vi "Parametri ADC.vi"() -> ()   [LabVIEW 2021]
uses:
  <vilib>/measure/madcrms.llb/Basic Averaged DC-RMS for 1 Chan.vi
  <vilib>/express/express analysis/Spectral/Block/exnSpectralBlock spectral measurements RMS poly.vi
  <vilib>/express/express analysis/Spectral/Block/exnSpectralBlock spectral measurements RMS DDT.vi
  <vilib>/express/express analysis/Spectral/XNode/ExpressSpectralMeasurementsBlockNode.xnode
  <vilib>/measure/NI_MAPro.lvlib
panel:
  out "Frequenza fondamentale":dbl
  out "ENOB ideale":dbl
  out "df":dbl
  out "Ampiezza fondamentale":dbl
  out "THD (db)":dbl
  out "ENOB (corretto rispetto al full scale)":dbl
  out "SINAD(db)":dbl
  out "SNR(db)":dbl
  out "DFT (dB)":dynamicdata(graph)
  out "numero punti dft":i32
  out "Ampiezza":dbl
  out "Frequenza":dbl
  out "SFDR":dbl
  out "DFT (lineare)":dynamicdata(graph)
  out "Segnale acquisito":dynamicdata(graph)
  # "distanza tra un punto\n della dft e il successivo"
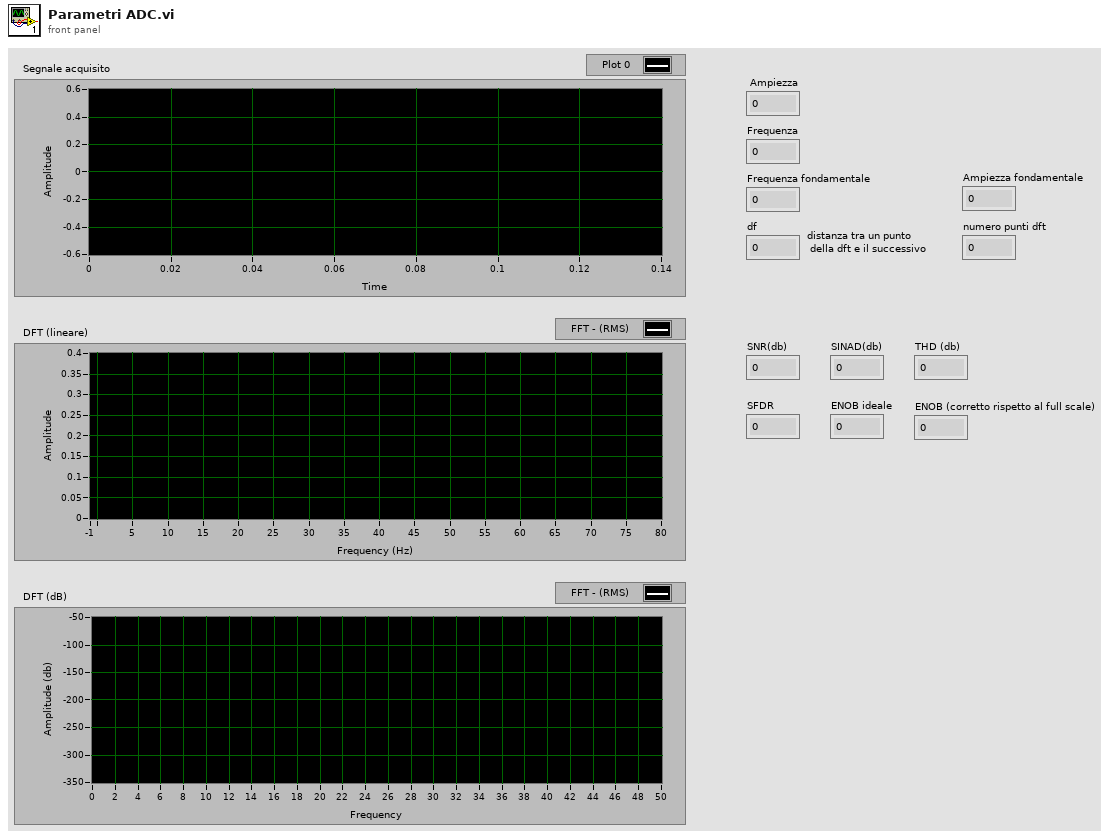
[diagram p1: front panel]
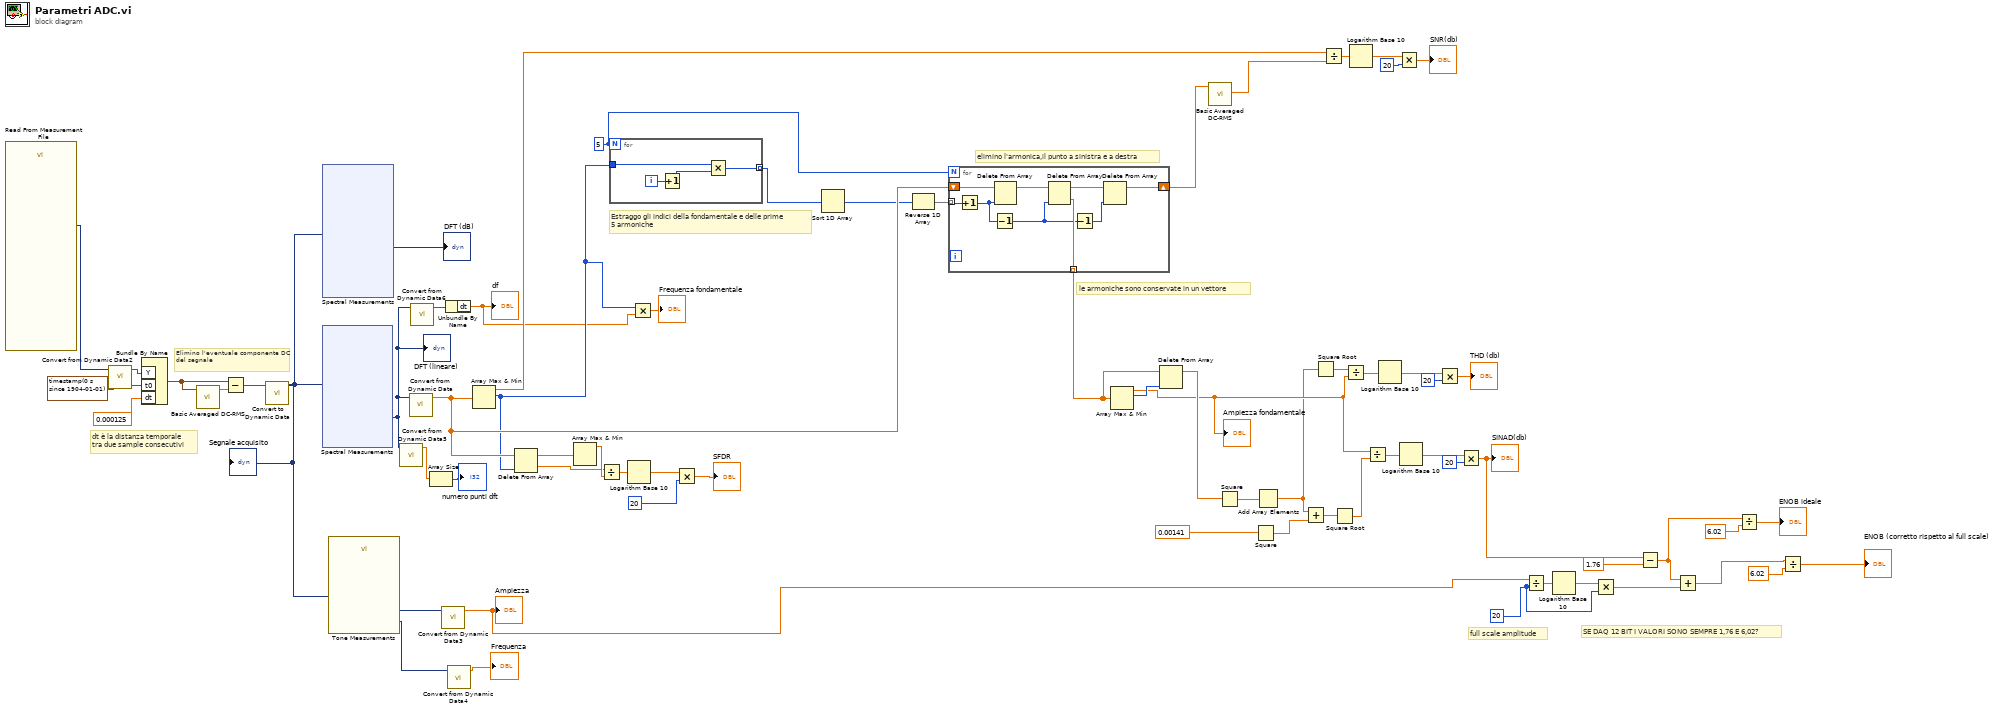
[diagram p0: block diagram]
diagram:
  w13 = 20
  w16 = 5
  # "Estraggo gli indici della fondamentale e delle prime\n5 armoniche"
  # "Elimino l'eventuale componente DC\ndel segnale"
  # "dt è la distanza temporale\ntra due sample consecutivi"
  # "SE DAQ 12 BIT I VALORI SONO SEMPRE 1,76 E 6,02?"
  # "le armoniche sono conservate in un vettore"
  # "elimino l'armonica,il punto a sinistra e a destra"
  # "full scale amplitude"
  n1 = call "Read From Measurement File"() -> ("Signals"=w8:dynamicdata)  [unwired: 6 in, 5 out]
  n2 = call "Convert from Dynamic Data2"("Dynamic Data Type"=w8) -> ("Waveform"=w69:waveform(dbl))  [unwired: 3 in]
  n3 = Bundle By Name("Y"=w69, "t0"=timestamp(0 s since 1904-01-01), "dt"=0.000125) -> (w4:waveform(dbl))  [unwired: 1 in]
  n4 = call-poly <vilib>:"Basic Averaged DC-RMS.vi"("signal in"=w4) -> ("DC value"=w3:dbl)  [unwired: 7 in, 3 out]
  n5 = Subtract(x=w4, y=w3) -> (x-y=w2:waveform(dbl))
  n6 = call "Convert to Dynamic Data"("Waveform"=w2) -> ("Dynamic Data Type"=w54:dynamicdata)  [unwired: 3 in]
  "Segnale acquisito" <- w54
  n7 = xnode "Spectral Measurements"("Signals"=w54) -> ("FFT - (RMS)"=w19:dynamicdata)  [unwired: 1 in, 2 out]
  "DFT (lineare)" <- w19
  n8 = xnode "Spectral Measurements"("Signals"=w54) -> ("FFT - (RMS)"=→"DFT (dB)":dynamicdata)  [unwired: 1 in, 2 out]
  n9 = call "Tone Measurements"("Signals"=w54) -> ("Frequency"=w57:dynamicdata, "Amplitude"=w58:dynamicdata)  [unwired: 8 in, 1 out]
  n10 = call "Convert from Dynamic Data5"("Dynamic Data Type"=w19) -> ("Array"=w56:dbl[])  [unwired: 3 in]
  n11 = call "Convert from Dynamic Data"("Dynamic Data Type"=w19) -> ("Array"=w52:dbl[])  [unwired: 3 in]
  n12 = call "Convert from Dynamic Data6"("Dynamic Data Type"=w19) -> ("Waveform"=w18:waveform(dbl))  [unwired: 3 in]
  n13 = Array Size(array=w56) -> (size(s)=→"numero punti dft":i32)
  n14 = call "Convert from Dynamic Data3"("Dynamic Data Type"=w58) -> ("Scalar"=w12:dbl)  [unwired: 3 in]
  "Ampiezza" <- w12
  n15 = Unbundle By Name(w18) -> ("dt"=w6:dbl)
  "df" <- w6
  n16 = call "Convert from Dynamic Data4"("Dynamic Data Type"=w57) -> ("Scalar"=→"Frequenza":dbl)  [unwired: 3 in]
  n17 = Array Max & Min(array=w52) -> (max value=w42:dbl, max index (indices)=w7:i32)  [unwired: 2 out]
  n18 = Delete From Array(array=w52, index=w7) -> (deleted portion=w61:dbl, array with subset deleted=w60:dbl[])  [unwired: 1 in]
  n19 = Array Max & Min(array=w60) -> (max value=w63:dbl)  [unwired: 3 out]
  n20 = Divide(x=w61, y=w63) -> (x/y=w64:dbl)
  n21 = for {
    N: w16 -> [_]
    tunnel: [w71] -> w17 mode=indexing
    tunnel: w7 -> [w70]
    i -> [w73]
    n22 = Increment(x=w73) -> (x+1=w72:i32)
    n23 = Multiply(x=w70, y=w72) -> (x*y=w71:i32)
  }
  n24 = Logarithm Base 10(1:w64) -> (0:w66:dbl)
  n25 = Multiply(x=w7, y=w6) -> (x*y=→"Frequenza fondamentale":dbl)
  n26 = Multiply(x=w66, y=20) -> (x*y=→"SFDR":dbl)
  n27 = Sort 1D Array(array=w17) -> (sorted array=w51:i32[])
  n28 = Reverse 1D Array(array=w51) -> (reversed array=w50:i32[])
  n29 = for {
    N: w16 -> [_]
    tunnel: w50 -> [w77] mode=indexing
    shift-right: [w79] -> w1
    shift-left: w52 -> [w82]
    tunnel: [w78] -> w48 mode=indexing
    n30 = Increment(x=w77) -> (x+1=w76:i32)
    n31 = Decrement(x=w76) -> (x-1=w75:i32)
    n32 = Delete From Array(array=w82, index=w76) -> (array with subset deleted=w81:dbl[])  [unwired: 1 in, 1 out]
    n33 = Delete From Array(array=w81, index=w75) -> (deleted portion=w78:dbl, array with subset deleted=w80:dbl[])  [unwired: 1 in]
    n34 = Decrement(x=w75) -> (x-1=w74:i32)
    n35 = Delete From Array(array=w80, index=w74) -> (array with subset deleted=w79:dbl[])  [unwired: 1 in, 1 out]
  }
  n36 = Array Max & Min(array=w48) -> (max value=w20:dbl, max index (indices)=w49:i32)  [unwired: 2 out]
  "Ampiezza fondamentale" <- w20
  n37 = Delete From Array(array=w48, index=w49) -> (array with subset deleted=w23:dbl[])  [unwired: 1 in, 1 out]
  n38 = call-poly <vilib>:"Basic Averaged DC-RMS.vi"("signal in"=w1) -> ("RMS value"=w44:dbl)  [unwired: 7 in, 3 out]
  n39 = Square(x=w23) -> (x^2=w24:dbl[])
  n40 = Square(x=0.00141) -> (x^2=w40:dbl)
  n41 = Add Array Elements(numeric array=w24) -> (sum=w14:dbl)
  n42 = Add(x=w14, y=w40) -> (x+y=w36:dbl)
  n43 = Square Root(x=w14) -> (sqrt(x)=w15:dbl)
  n44 = Divide(x=w42, y=w44) -> (x/y=w45:dbl)
  n45 = Square Root(x=w36) -> (sqrt(x)=w35:dbl)
  n46 = Divide(x=w15, y=w20) -> (x/y=w26:dbl)
  n47 = Logarithm Base 10(1:w45) -> (0:w47:dbl)
  n48 = Divide(x=w20, y=w35) -> (x/y=w37:dbl)
  n49 = Logarithm Base 10(1:w26) -> (0:w28:dbl)
  n50 = Multiply(x=w47, y=20) -> (x*y=→"SNR(db)":dbl)
  n51 = Logarithm Base 10(1:w37) -> (0:w39:dbl)
  n52 = Multiply(x=w28, y=20) -> (x*y=→"THD (db)":dbl)
  n53 = Multiply(x=w39, y=20) -> (x*y=w29:dbl)
  "SINAD(db)" <- w29
  n54 = Divide(x=w12, y=w13) -> (x/y=w33:dbl)
  n55 = Logarithm Base 10(1:w33) -> (0:w34:dbl)
  n56 = Multiply(x=w34, y=w13) -> (x*y=w32:dbl)
  n57 = Subtract(x=w29, y=1.76 ("x")) -> (x-y=w10:dbl)
  n58 = Add(x=w10, y=w32) -> (x+y=w21:dbl)
  n59 = Divide(x=w10, y=6.02) -> (x/y=→"ENOB ideale":dbl)
  n60 = Divide(x=w21, y=6.02) -> (x/y=→"ENOB (corretto rispetto al full scale)":dbl)
